vi "$CNXN_DataQ_2Ch.vi"() -> ()   [LabVIEW 2024]
doc: "This example performs writes and reads on a serial port, as directed by the user. You can press the Write and Read buttons, and change the Read Count, while the example is running.\n\nThe parameters set for the serial port must match the parameters of the connected instrument or device. In this example, the Read Count parameter specifies the number of bytes that the serial port reads. If there were more bytes at the port than the specified number, those bytes would not be read. If there were less bytes at the port than the specified number, you would receive a timeout error.\n\nThis example expands upon the flow control options for XON and XOFF, allowing the user to choose those control characters. Also, the user can enable or disable a termination character. Some devices require a termination character in order to identify the end of command strings. Some devices send a termination character to signify the end of data to be read. This example shows how you can end the Read operation once a termination character is detected in the buffer and/or append a termination character at the end of the Write data."
uses:
  <vilib>/Instr/_visa.llb/VISA Configure Serial Port (Instr).vi
panel:
  out "Read Buffer":string
  out "Waveform Chart":dbl[][](graph)=[[1.71783447265625, 1.72332763671875], [1.71722412109375, 1.72210693359375], [1.71295166015625, 1.7242431640625], [1.70684814453125, 1.7236328125], [1.7156982421875, 1.72454833984375], [1.7193603515625, 1.72607421875], [1.70989990234375, 1.7266845703125], [1.71478271484375, 1.72576904296875], [1.71539306640625, 1.72088623046875], [1.71844482421875, 1.7230224609375], [1.717529296875, 1.72576904296875], [1.71844482421875, 1.72576904296875], [1.71234130859375, 1.72454833984375], [1.71905517578125, 1.72607421875], [1.71630859375, 1.724853515625], [1.71539306640625, 1.71783447265625], [1.71844482421875, 1.72393798828125], [1.71630859375, 1.72882080078125], [1.71356201171875, 1.72882080078125], [1.71173095703125, 1.72698974609375], [1.719970703125, 1.72515869140625], [1.71875, 1.72454833984375], [1.715087890625, 1.72454833984375], [1.71417236328125, 1.7266845703125], [1.719970703125, 1.724853515625], [1.71539306640625, 1.72210693359375], [1.719970703125, 1.72515869140625], [1.70745849609375, 1.7230224609375], [1.71539306640625, 1.72698974609375], [1.71875, 1.7254638671875], [1.71630859375, 1.72607421875], [1.71539306640625, 1.72698974609375], [1.71539306640625, 1.7242431640625], [1.719970703125, 1.72332763671875], [1.7181396484375, 1.72943115234375], [1.71417236328125, 1.727294921875], [1.717529296875, 1.72607421875], [1.715087890625, 1.7266845703125], [1.7138671875, 1.72515869140625], [1.715087890625, 1.72607421875], [1.7169189453125, 1.727294921875], [1.71722412109375, 1.73004150390625], [1.71234130859375, 1.727294921875], [1.71630859375, 1.72454833984375], [1.71173095703125, 1.72760009765625], [1.72210693359375, 1.72607421875], [1.7181396484375, 1.7254638671875], [1.71539306640625, 1.72943115234375], [1.71295166015625, 1.727294921875], [1.71539306640625, 1.72943115234375], [1.708984375, 1.7254638671875], [1.7156982421875, 1.724853515625], [1.71722412109375, 1.72088623046875], [1.7181396484375, 1.7236328125], [1.71875, 1.72271728515625], [1.71661376953125, 1.724853515625], [1.71630859375, 1.72607421875], [1.7144775390625, 1.72760009765625], [1.71722412109375, 1.72515869140625], [1.7156982421875, 1.728515625], [1.717529296875, 1.72119140625], [1.715087890625, 1.7242431640625], [1.7169189453125, 1.72576904296875], [1.71478271484375, 1.72607421875], [1.719970703125, 1.72607421875], [1.71875, 1.727294921875], [1.71783447265625, 1.727294921875], [1.71722412109375, 1.72607421875], [1.71783447265625, 1.728515625], [1.71661376953125, 1.7279052734375], [1.7193603515625, 1.72698974609375], [1.71539306640625, 1.7236328125], [1.71630859375, 1.7236328125], [1.7138671875, 1.72271728515625], [1.72088623046875, 1.7242431640625], [1.7169189453125, 1.72760009765625], [1.7156982421875, 1.72119140625], [1.70806884765625, 1.7230224609375], [1.712646484375, 1.72698974609375], [1.71112060546875, 1.7254638671875], [1.71844482421875, 1.72698974609375], [1.717529296875, 1.7279052734375], [1.722412109375, 1.72607421875], [1.72210693359375, 1.72698974609375], [1.71875, 1.72515869140625], [1.7205810546875, 1.7242431640625], [1.71905517578125, 1.72576904296875], [1.71630859375, 1.7254638671875], [1.7169189453125, 1.72760009765625], [1.7156982421875, 1.72698974609375], [1.71234130859375, 1.727294921875], [1.7169189453125, 1.72607421875], [1.71722412109375, 1.72607421875], [1.71722412109375, 1.72698974609375], [1.71630859375, 1.71844482421875], [1.7156982421875, 1.72271728515625], [1.71234130859375, 1.7236328125], [1.71295166015625, 1.72454833984375], [1.71661376953125, 1.72515869140625], [1.71630859375, 1.72698974609375], [1.71630859375, 1.7254638671875], [1.7120361328125, 1.7254638671875], [1.71112060546875, 1.72515869140625], [1.71630859375, 1.724853515625], [1.7156982421875, 1.72119140625], [1.71234130859375, 1.7279052734375], [1.71356201171875, 1.7279052734375], [1.71356201171875, 1.7230224609375], [1.715087890625, 1.7303466796875], [1.7138671875, 1.72271728515625], [1.71722412109375, 1.72576904296875], [1.71356201171875, 1.7230224609375], [1.7132568359375, 1.72943115234375], [1.71844482421875, 1.72882080078125], [1.71478271484375, 1.72698974609375], [1.7144775390625, 1.72607421875], [1.719970703125, 1.72698974609375], [1.7236328125, 1.72393798828125], [1.71875, 1.71966552734375], [1.722412109375, 1.72576904296875], [1.7315673828125, 1.7236328125], [1.71783447265625, 1.72515869140625], [1.7144775390625, 1.72454833984375], [1.71356201171875, 1.728515625], [1.71356201171875, 1.72698974609375], [1.719970703125, 1.72454833984375], [1.71905517578125, 1.72515869140625], [1.71722412109375, 1.7242431640625], [1.71539306640625, 1.71478271484375], [1.7156982421875, 1.72698974609375], [1.7193603515625, 1.72607421875], [1.71630859375, 1.72943115234375], [1.7156982421875, 1.73004150390625], [1.71295166015625, 1.7242431640625], [1.7144775390625, 1.7242431640625], [1.71417236328125, 1.72454833984375], [1.7156982421875, 1.72515869140625], [1.71783447265625, 1.7254638671875], [1.71722412109375, 1.7279052734375], [1.71783447265625, 1.7279052734375], [1.71661376953125, 1.728515625], [1.71722412109375, 1.7254638671875], [1.715087890625, 1.72515869140625], [1.71630859375, 1.72027587890625], [1.71844482421875, 1.72149658203125], [1.71844482421875, 1.7205810546875], [1.71630859375, 1.72821044921875], [1.71539306640625, 1.728515625], [1.71417236328125, 1.7254638671875], [1.7144775390625, 1.728515625], [1.71722412109375, 1.7254638671875], [1.7181396484375, 1.72698974609375], [1.72119140625, 1.724853515625], [1.71539306640625, 1.728515625], [1.7144775390625, 1.72515869140625], [1.71630859375, 1.72698974609375], [1.7169189453125, 1.72393798828125], [1.71630859375, 1.72698974609375], [1.71539306640625, 1.72698974609375], [1.7144775390625, 1.72393798828125], [1.712646484375, 1.72515869140625], [1.71173095703125, 1.7236328125], [1.719970703125, 1.72515869140625], [1.7138671875, 1.7254638671875], [1.71417236328125, 1.728515625], [1.7120361328125, 1.7279052734375], [1.7169189453125, 1.72576904296875], [1.71417236328125, 1.7230224609375], [1.715087890625, 1.72576904296875], [1.7144775390625, 1.72576904296875], [1.71783447265625, 1.72393798828125], [1.715087890625, 1.72821044921875], [1.71356201171875, 1.7254638671875], [1.7156982421875, 1.72698974609375], [1.71295166015625, 1.72454833984375], [1.7169189453125, 1.7279052734375]]
  in  "Command List":string="stop\nencode 0\nslist 0 0\nslist 1 1\nsrate 6000\nps 2\ndec 1\ndeca 3\nnop\n"
  in  "Stop":bool
  in  "2108 CDC Virtual COM":refnum<visa-resource-name>="COM3"
  # "ASRL4::INSTR"
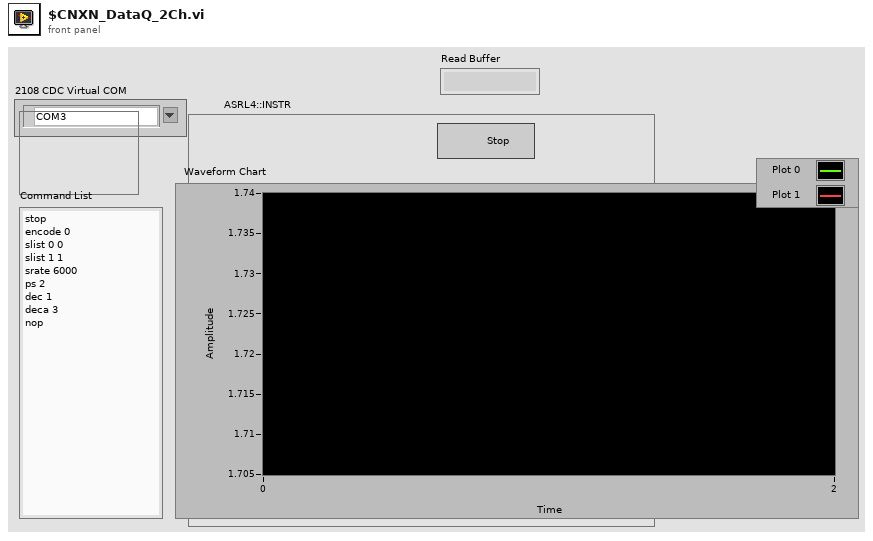
[diagram p1: front panel]
types:
  T1 = enum16{"big-endian, network order", "native, host order", "little-endian"}
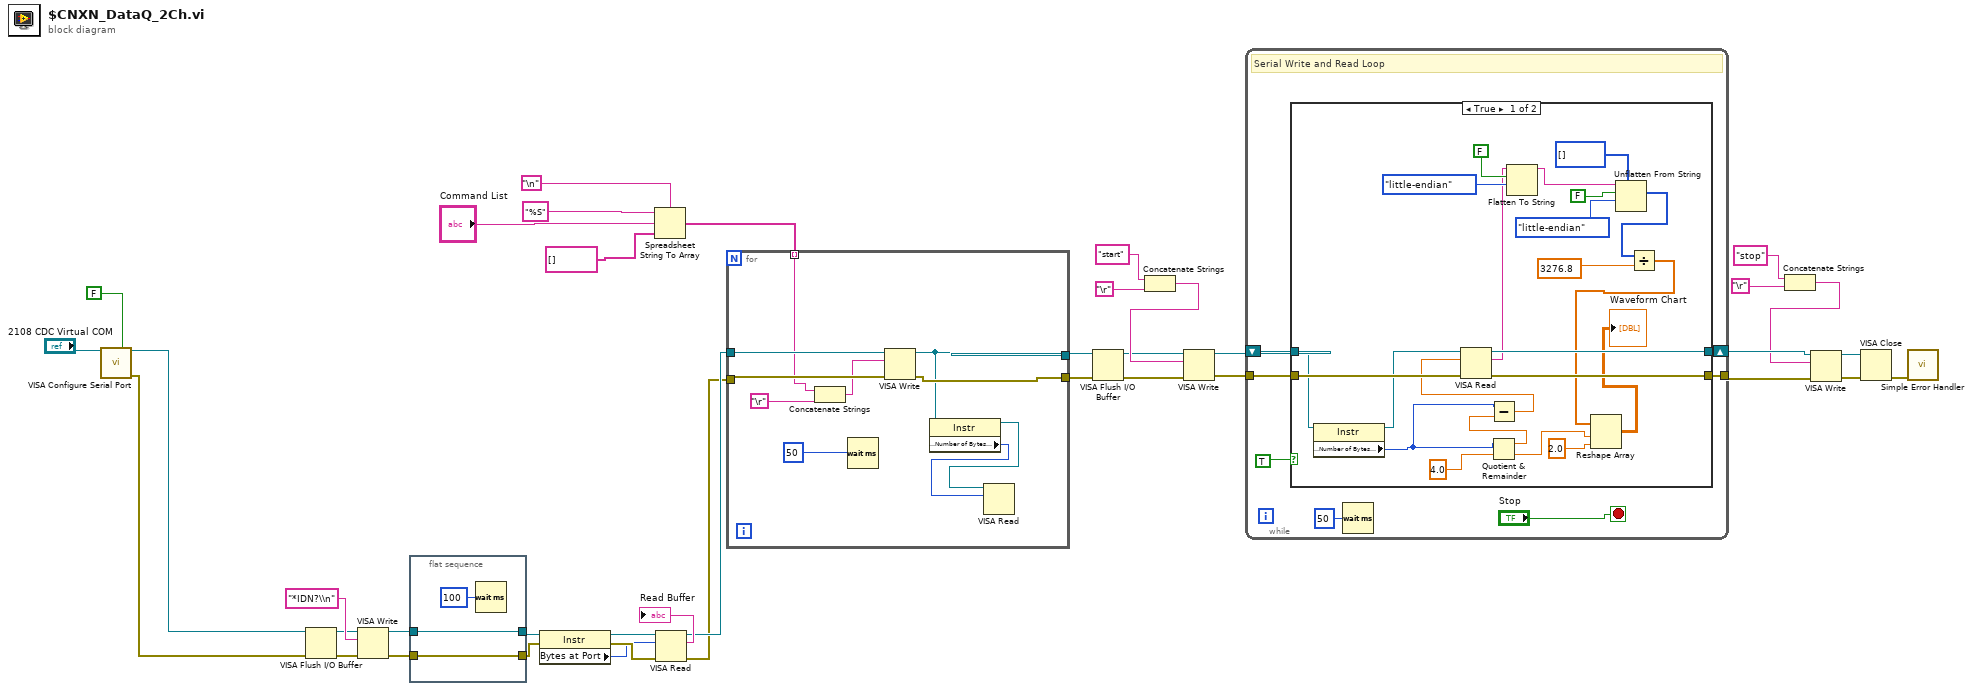
[diagram p0: block diagram]
diagram:
  n1 = call-poly "VISA Configure Serial Port"("VISA resource name"="2108 CDC Virtual COM", "Enable Termination\nChar (T)"=FALSE) -> ("VISA resource name out"=w2:refnum<visa-resource-name>, "error out"=w1:errorcluster)  [unwired: 8 in, 4 out]
  n2 = VISA Flush I/O Buffer(VISA resource name=w2, error in (no error)=w1) -> (VISA resource name out=w4:refnum<visa-resource-name>, error out=w3:errorcluster)  [unwired: 1 in]
  n3 = VISA Write(VISA resource name=w4, write buffer="*IDN?\\n", error in (no error)=w3) -> (VISA resource name out=w10:refnum<visa-resource-name>, error out=w15:errorcluster)  [unwired: 1 out]
  n4 = flat-sequence {
    tunnel: w10 -> [w41]
    tunnel: [w41] -> w13
    tunnel: w15 -> [w40]
    tunnel: [w40] -> w12
    frame #0 {
      n5 = Wait (ms)(milliseconds to wait=u32 100) -> ()  [unwired: 1 out]
    }
  }
  n6 = property class="Instr"(reference=w13, error in=w12) -> (reference out=w8:refnum<visa-resource-name>, error out=w11:errorcluster, "Bytes at Port"=w9:u32)
  n7 = Spreadsheet String To Array(delimiter (Tab)="\n", format string="%S", spreadsheet string="Command List", array type (2D Dbl)=string[] []) -> (array=w35:string[])
  n8 = VISA Read(VISA resource name=w8, byte count=w9, error in (no error)=w11) -> (VISA resource name out=w6:refnum<visa-resource-name>, read buffer=→"Read Buffer":string, error out=w5:errorcluster)  [unwired: 1 out]
  n9 = for {
    tunnel: w35 -> [w49] mode=indexing
    tunnel: w6 -> [w52]
    tunnel: w5 -> [w51]
    tunnel: [w45] -> w19
    tunnel: [w46] -> w17
    n10 = Concatenate Strings(w49, "\r") -> (w47:string)
    n11 = Wait (ms)(milliseconds to wait=u32 50) -> ()  [unwired: 1 out]
    n12 = VISA Write(VISA resource name=w52, write buffer=w47, error in (no error)=w51) -> (VISA resource name out=w45:refnum<visa-resource-name>, error out=w46:errorcluster)  [unwired: 1 out]
    n13 = property class="Instr"(reference=w45) -> (reference out=w44:refnum<visa-resource-name>, "Serial Settings:Number of Bytes at Serial Port"=w43:u32)  [unwired: 1 in, 1 out]
    n14 = VISA Read(VISA resource name=w44, byte count=w43) -> ()  [unwired: 1 in, 4 out]
  }
  n15 = VISA Flush I/O Buffer(VISA resource name=w19, error in (no error)=w17) -> (VISA resource name out=w18:refnum<visa-resource-name>, error out=w16:errorcluster)  [unwired: 1 in]
  n16 = Concatenate Strings("start", "\r") -> (w23:string)
  n17 = VISA Write(VISA resource name=w18, write buffer=w23, error in (no error)=w16) -> (VISA resource name out=w22:refnum<visa-resource-name>, error out=w21:errorcluster)  [unwired: 1 out]
  n18 = while {
    shift-right: [w59] -> w32
    shift-left: w22 -> [w55]
    tunnel: w21 -> [w54]
    tunnel: [w57] -> w29
    stop <- "Stop" stop-if-true
    # "Serial Write and Read Loop"
    n19 = case shown="True" TRUE {
      tunnel: [w80 w83] -> w59
      tunnel: w55 -> [w78 w83]
      tunnel: w54 -> [w81 w82]
      tunnel: [w73 w82] -> w57
      frame True {
        n20 = property class="Instr"(reference=w78) -> (reference out=w72:refnum<visa-resource-name>, "Serial Settings:Number of Bytes at Serial Port"=w77:u32)  [unwired: 1 in, 1 out]
        n21 = Quotient & Remainder(x=w77, y=4.0) -> (x-y*floor(x/y)=w75:dbl, floor(x/y)=w61:dbl)
        n22 = Subtract(x=w77, y=w75) -> (x-y=w74:dbl)
        n23 = VISA Read(VISA resource name=w72, byte count=w74, error in (no error)=w81) -> (VISA resource name out=w80:refnum<visa-resource-name>, read buffer=w66:string, error out=w73:errorcluster)  [unwired: 1 out]
        n24 = Flatten To String(anything=w66, prepend array or string size? (T)=FALSE, byte order (0:big-endian, network order)=T1."little-endian") -> (data string=w67:string)  [unwired: 1 in, 2 out]
        n25 = Unflatten From String(type=i16[] [], binary string=w67, data includes array or string size? (T)=FALSE, byte order (0:big-endian, network order)=T1."little-endian") -> (value=w65:i16[])  [unwired: 1 in, 2 out]
        n26 = Divide(x=w65, y=3276.8) -> (x/y=w63:dbl[])
        n27 = Reshape Array(w63, w61, 2.0) -> (→"Waveform Chart":dbl[][])
      }
      frame False {
      }
    }
    n28 = Wait (ms)(milliseconds to wait=u32 50) -> ()  [unwired: 1 out]
  }
  n29 = Concatenate Strings("stop", "\r") -> (w26:string)
  n30 = VISA Write(VISA resource name=w32, write buffer=w26, error in (no error)=w29) -> (VISA resource name out=w31:refnum<visa-resource-name>, error out=w30:errorcluster)  [unwired: 1 out]
  n31 = VISA Close(VISA resource name=w31, error in (no error)=w30) -> (error out=w39:errorcluster)
  n32 = call <vilib>:"Simple Error Handler.vi"("error in (no error)"=w39) -> ()  [unwired: 1 in, 8 out]
